vi "Generate Sine Waves 120 degree phase difference.vi"(4 "sampling info":cluster{"Fs":dbl, "#s":dbl}, 6 "Signal Data":cluster{"f":dbl, "startPhase":dbl, "dPhase":dbl}={"f"=1000.0, "startPhase"=0.0, "dPhase"=0.0}, 8 "error in (no error)":errorcluster, 11 "channels":string) -> (0 "error out":errorcluster, 3 "signal out":waveform(dbl))   [LabVIEW 2024]
uses:
  <vilib>/measure/NI_MABase.lvlib
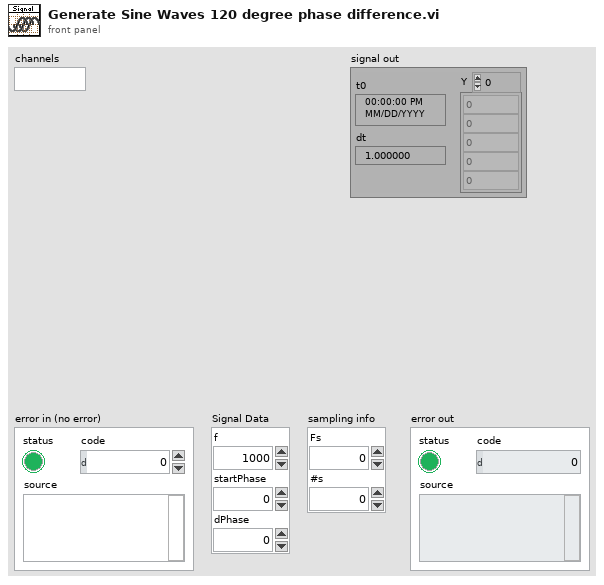
[diagram p1: front panel]
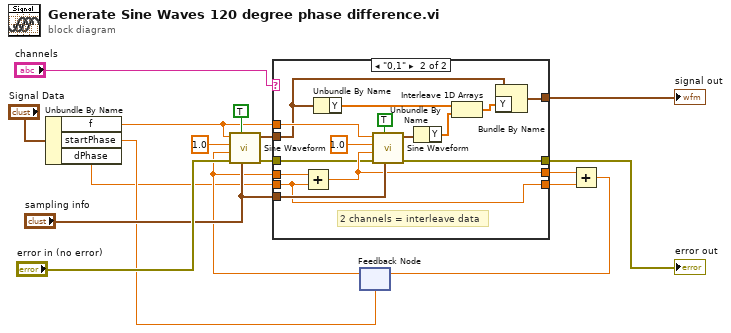
[diagram p0: block diagram]
diagram:
  n1 = Unbundle By Name("Signal Data") -> ("f"=w4:dbl, "startPhase"=w3:dbl, "dPhase"=w2:dbl)
  n2 = feedback #1(w3) -> (w7:dbl)
  n3 = call <vilib>:"Sine Waveform.vi"("sampling info"="sampling info", "reset signal"=TRUE, "error in (no error)"="error in (no error)", "phase"=w7, "amplitude"=1.0, "frequency"=w4) -> ("error out"=w13:errorcluster, "signal out"=w15:waveform(dbl))  [unwired: 4 in]
  n4 = case shown="\"0,1\"" "channels" {
    tunnel: w4 -> [_ w36]
    tunnel: "sampling info" -> [_ w35]
    tunnel: w7 -> [w19 w34]
    tunnel: [w19 w33] -> w9
    tunnel: w13 -> [w20 w31]
    tunnel: w15 -> [w21 w23]
    tunnel: [w20 w29] -> w16
    tunnel: [w21 w27] -> w17
    tunnel: w2 -> [w18 w22]
    tunnel: [w18 w22] -> w1
    frame "0", Default {
      # "1 channel"
    }
    frame "0,1" {
      # "2 channels = interleave data"
      n5 = Add(x=w34, y=w22) -> (x+y=w33:dbl)
      n6 = Unbundle By Name(w23) -> ("Y"=w26:dbl[])
      n7 = call <vilib>:"Sine Waveform.vi"("sampling info"=w35, "reset signal"=TRUE, "error in (no error)"=w31, "phase"=w33, "amplitude"=1.0, "frequency"=w36) -> ("error out"=w29:errorcluster, "signal out"=w28:waveform(dbl))  [unwired: 4 in]
      n8 = Unbundle By Name(w28) -> ("Y"=w25:dbl[])
      n9 = Interleave 1D Arrays(w26, w25) -> (w24:dbl[])
      n10 = Bundle By Name(cluster=w23, "Y"=w24) -> (w27:waveform(dbl))
    }
  }
  "signal out" <- w17
  "error out" <- w16
  n11 = Add(x=w9, y=w1) -> (x+y=w6:dbl)
  n12 = feedback-in #1(w6) -> ()
